vi "GEN_WriteStatus.vi"(7 "Input String":string, 8 "error in (no error)":errorcluster, 10 "Config_Cluster":T3={"Hardware"={"Measure Rate (1/s)"=0, "HP DMM VISA"="", "LS 335 VISA"="", "HP DM"={"Range"=enum."Autorange", "Autozero"=FALSE, "Display"=enum."3 1/2 Digit", "Blank LCD"=FALSE}}, "Operation"={"Operation Mode"=enum."Idle-Off", "Status"="", "NewLog?"=FALSE, "OvenWarn"=FALSE}}, 11 "Status Ref":refnum<vi>) -> (0 "error out":errorcluster, 2 "Config_Cluster Out":T1={"General"={"Config.ini"=path "", "Default Logging Path"=path ""}, "Hardware"={"Measure Rate (1/s)"=0, "HP DMM VISA"="", "LS 335 VISA"="", "HP DM"={"Range"=enum."Autorange", "Autozero"=FALSE, "Display"=enum."3 1/2 Digit", "Blank LCD"=FALSE}}, "Operation"={"Operation Mode"=enum."Idle-Off", "Status"="", "NewLog?"=FALSE, "OvenWarn"=FALSE}})   [LabVIEW 2021]
uses:
  Mode_Enum.ctl
  Config_Cluster.ctl
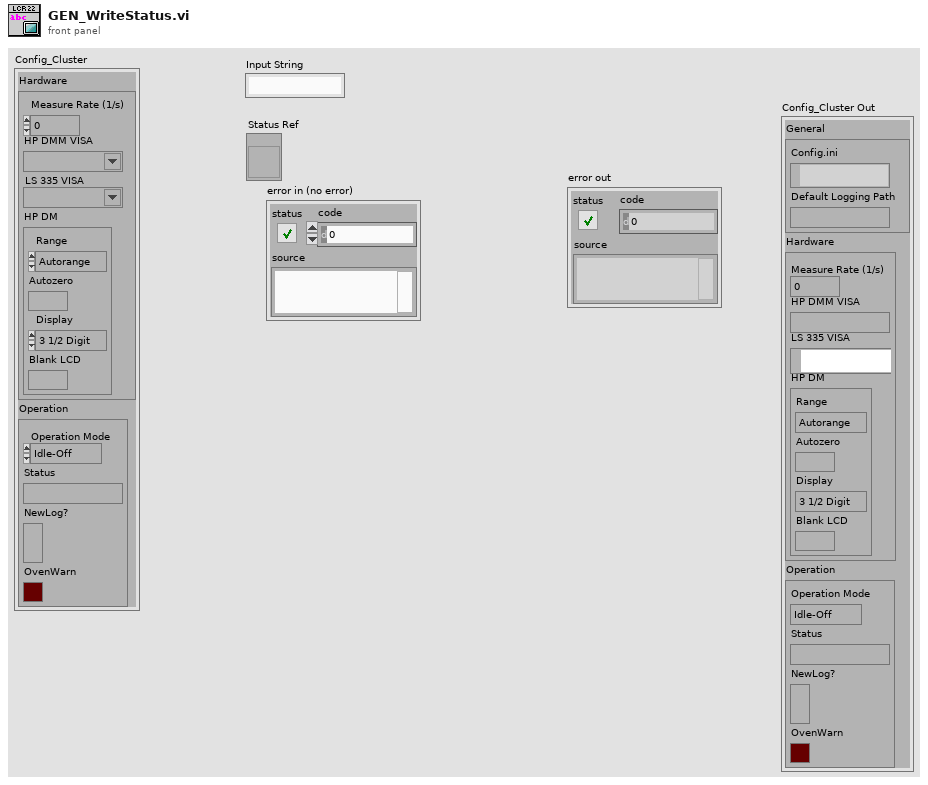
[diagram p1: front panel]
types:
  T1 = typedef "Config_Cluster.ctl" = cluster{"General":cluster{"Config.ini":path, "Default Logging Path":path}, "Hardware":cluster{"Measure Rate (1/s)":i32, "HP DMM VISA":refnum<visa-resource-name>, "LS 335 VISA":refnum<visa-resource-name>, "HP DM":cluster{"Range":enum16{"Autorange", "30mV", "300mV", "3V", "30V"}, "Autozero":bool, "Display":enum16{"3 1/2 Digit", "4 1/2 Digit", "5 1/2 Digit"}, "Blank LCD":bool}}, "Operation":cluster{"Operation Mode":T2, "Status":string, "NewLog?":bool, "OvenWarn":bool}}
  T2 = typedef "Mode_Enum.ctl" = enum16{"OvenNRDY", "Logging", "Idle-Off", "Idle"}
  T3 = typedef "Config_Cluster.ctl" = cluster{"Hardware":cluster{"Measure Rate (1/s)":i32, "HP DMM VISA":refnum<visa-resource-name>, "LS 335 VISA":refnum<visa-resource-name>, "HP DM":cluster{"Range":enum16{"Autorange", "30mV", "300mV", "3V", "30V"}, "Autozero":bool, "Display":enum16{"3 1/2 Digit", "4 1/2 Digit", "5 1/2 Digit"}, "Blank LCD":bool}}, "Operation":cluster{"Operation Mode":T2, "Status":string, "NewLog?":bool, "OvenWarn":bool}}
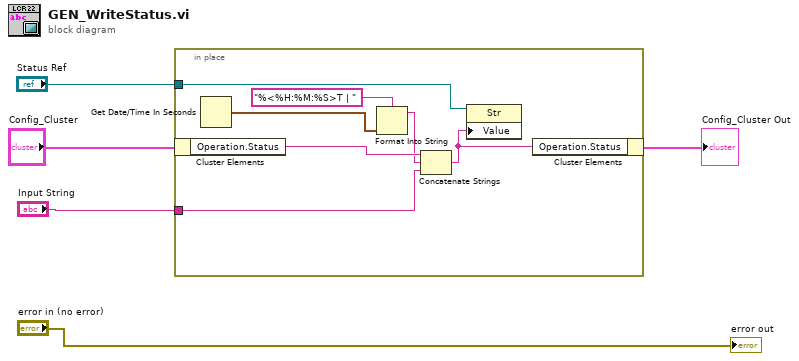
[diagram p0: block diagram]
diagram:
  n1 = in-place {
    in-place-border: "Input String" -> [w7]
    in-place-border: "Status Ref" -> [w11]
    n2 = in-place-cluster #1("Config_Cluster") -> ("Operation.Status"=w12:string)
    n3 = Get Date/Time In Seconds() -> (seconds since 1Jan1904=w9:timestamp)
    n4 = Format Into String(format string="%<%H:%M:%S>T | ", w9) -> (resulting string=w6:string)  [unwired: 2 in, 1 out]
    n5 = Concatenate Strings(w12, w6, w7) -> (w10:string)
    n6 = property class="Str"(reference=w11, "Value"=w10) -> ()  [unwired: 1 in, 2 out]
    n7 = in-place-cluster #1("Operation.Status"=w10) -> (→"Config_Cluster Out":T3)
  }
  "error out" <- "error in (no error)"
